vi "Process LLBs.vi"(8 "error in (no error)":errorcluster {"code" format="Error %.0f"}, 10 "LLBs":refnum<class "LLB Documentation.lvclass">[](array[class]), 11 "VIDoc Printer In":refnum<class "VIDoc Printer.lvclass">) -> (0 "error out":errorcluster {"code" format="Error %.0f"}, 3 "VIDoc Printer Out":refnum<class "VIDoc Printer.lvclass">)   [LabVIEW 2023, in "VIDoc Printer.lvlib" / "VIDoc Printer.lvclass"]
uses:
  VIDoc Printer.lvclass
  VIDoc Printer.lvclass/VIDoc Printer.ctl
  Parsing/LLB Documentation/LLB Documentation.lvclass
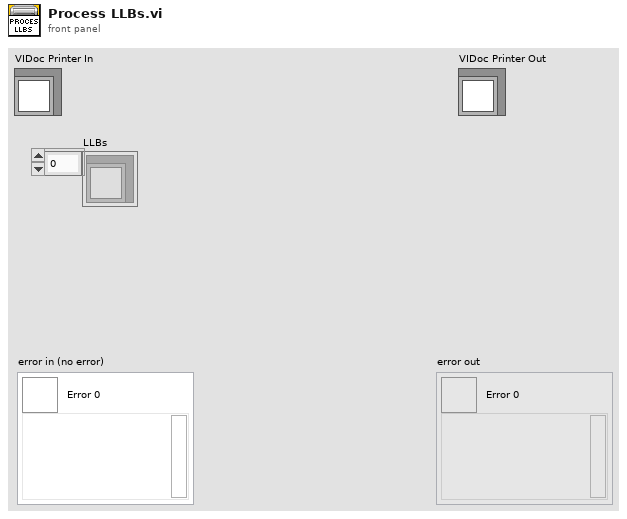
[diagram p1: front panel]
types:
  T1 = typedef "VIDoc Printer.lvlib/VIDoc Printer.lvclass/Process LLB Enum.ctl" = enum16{"Header", "By List", "Methods", "Controls"}
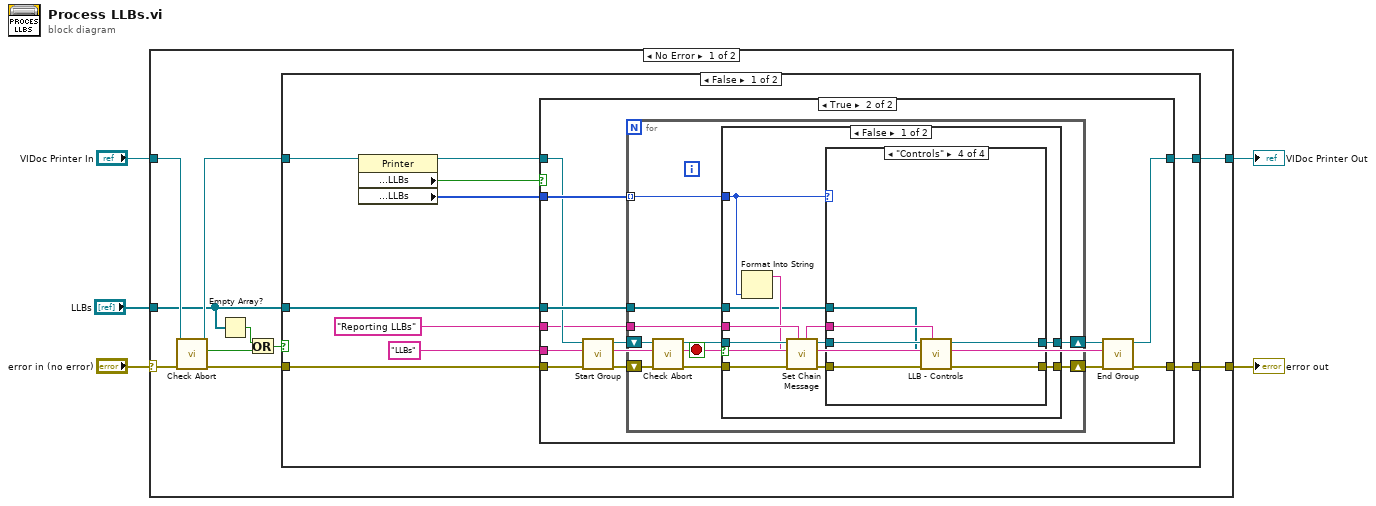
[diagram p0: block diagram]
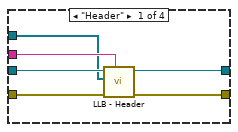
[diagram p3: hidden frame]
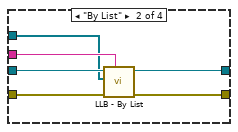
[diagram p4: hidden frame]
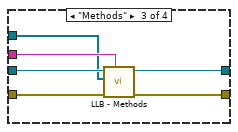
[diagram p5: hidden frame]
diagram:
  n1 = case shown="No Error" "error in (no error)" {
    selector: "error in (no error)" -> [w15 w90]
    tunnel: [w10 w90] -> w4
    tunnel: [w9 w89] -> w2
    tunnel: "VIDoc Printer In" -> [w12 w89]
    tunnel: "LLBs" -> [w8 _]
    frame No Error {
      n2 = call "Check Abort.vi"("error in (no error)"=w15, "VIDoc Printer In"=w12) -> ("error out"=w14:errorcluster, "Abort?"=w11:bool, "VIDoc Printer Out"=w13:refnum<class "VIDoc Printer.lvclass">)  [unwired: 7 in]
      n3 = Empty Array?(array=w8) -> (empty?=w6:bool)
      n4 = Or(x=w6, y=w11) -> (x .or. y?=w7:bool)
      n5 = case shown="False" w7 {
        tunnel: w8 -> [w25 _]
        tunnel: w14 -> [w22 w88]
        tunnel: w13 -> [w23 w87]
        tunnel: [w20 w88] -> w10
        tunnel: [w21 w87] -> w9
        frame False {
          n6 = property class="Printer"(reference=w23) -> (reference out=w24:refnum<class "VIDoc Printer.lvclass">, "Properties:Settings:Enabled Sections:LLBs"=w19:bool, "Properties:Process Lists:LLBs"=w18:T1[])  [unwired: 1 in, 1 out]
          n7 = case shown="True" w19 {
            tunnel: w22 -> [w27 w37]
            tunnel: "Reporting LLBs" ("string") -> [_ w29]
            tunnel: [w27 w30] -> w20
            tunnel: w25 -> [_ w39]
            tunnel: w24 -> [w26 w34]
            tunnel: [w26 w31] -> w21
            tunnel: w18 -> [_ w38]
            tunnel: "LLBs" -> [_ w28]
            frame False {
            }
            frame True {
              n8 = call-dynamic "Start Group.vi"("error in (no error)"=w37, "Group"=w28, "VIDoc Printer In"=w34) -> ("error out"=w36:errorcluster, "VIDoc Printer Out"=w35:refnum<class "VIDoc Printer.lvclass">)  [unwired: 7 in]
              n9 = for {
                shift-right: [w47] -> w32
                shift-left: w36 -> [w49]
                tunnel: w29 -> [w43]
                tunnel: w39 -> [w42]
                shift-right: [w45] -> w33
                shift-left: w35 -> [w48]
                tunnel: w38 -> [w41] mode=indexing
                stop <- w40 stop-if-true
                n10 = call "Check Abort.vi"("error in (no error)"=w49, "VIDoc Printer In"=w48) -> ("error out"=w46:errorcluster, "Abort?"=w40:bool, "VIDoc Printer Out"=w44:refnum<class "VIDoc Printer.lvclass">)  [unwired: 7 in]
                n11 = case shown="False" w40 {
                  tunnel: [w60 w86] -> w47
                  tunnel: w46 -> [w57 w86]
                  tunnel: [w59 w85] -> w45
                  tunnel: w44 -> [w55 w85]
                  tunnel: w43 -> [w54 _]
                  tunnel: w42 -> [w51 _]
                  tunnel: w41 -> [w53 _]
                  frame False {
                    n12 = Format Into String(w53) -> (resulting string=w52:string)  [unwired: 3 in, 1 out]
                    n13 = call "Set Chain Message.vi"("Msg Chain"=w54, "error in (no error)"=w57, "New"=w52, "VIDoc Printer In"=w55) -> ("error out"=w58:errorcluster, "VIDoc Printer Out"=w56:refnum<class "VIDoc Printer.lvclass">, "Msg Chain out"=w50:string)  [unwired: 5 in]
                    n14 = case shown="\"Controls\"" w53 {
                      tunnel: w58 -> [w65 w71 w77 w83]
                      tunnel: [w63 w69 w75 w81] -> w60
                      tunnel: w56 -> [w66 w72 w78 w84]
                      tunnel: [w64 w70 w76 w82] -> w59
                      tunnel: w51 -> [w61 w67 w73 w79]
                      tunnel: w50 -> [w62 w68 w74 w80]
                      frame "Header" {
                        n15 = call-dynamic "LLB - Header.vi"("Msg Chain"=w62, "error in (no error)"=w65, "LLBs"=w61, "VIDoc Printer In"=w66) -> ("error out"=w63:errorcluster, "VIDoc Printer Out"=w64:refnum<class "VIDoc Printer.lvclass">)  [unwired: 6 in]
                      }
                      frame "By List" {
                        n16 = call-dynamic "LLB - By List.vi"("Msg Chain"=w68, "error in (no error)"=w71, "LLBs"=w67, "VIDoc Printer In"=w72) -> ("error out"=w69:errorcluster, "VIDoc Printer Out"=w70:refnum<class "VIDoc Printer.lvclass">)  [unwired: 6 in]
                      }
                      frame "Methods" {
                        n17 = call-dynamic "LLB - Methods.vi"("Msg Chain"=w74, "error in (no error)"=w77, "LLBs"=w73, "VIDoc Printer In"=w78) -> ("error out"=w75:errorcluster, "VIDoc Printer Out"=w76:refnum<class "VIDoc Printer.lvclass">)  [unwired: 6 in]
                      }
                      frame "Controls" {
                        n18 = call-dynamic "LLB - Controls.vi"("Msg Chain"=w80, "error in (no error)"=w83, "LLBs"=w79, "VIDoc Printer In"=w84) -> ("error out"=w81:errorcluster, "VIDoc Printer Out"=w82:refnum<class "VIDoc Printer.lvclass">)  [unwired: 6 in]
                      }
                    }
                  }
                  frame True {
                  }
                }
              }
              n19 = call-dynamic "End Group.vi"("error in (no error)"=w32, "Group"=w28, "VIDoc Printer In"=w33) -> ("error out"=w30:errorcluster, "VIDoc Printer Out"=w31:refnum<class "VIDoc Printer.lvclass">)  [unwired: 7 in]
            }
          }
        }
        frame True {
        }
      }
    }
    frame Error {
    }
  }
  "error out" <- w4
  "VIDoc Printer Out" <- w2
